vi "限幅器（Path）.vi"(3 "下限":path, 4 "X_in":path, 5 "上限":path) -> (1 "X_Out":path)   [LabVIEW 2012]
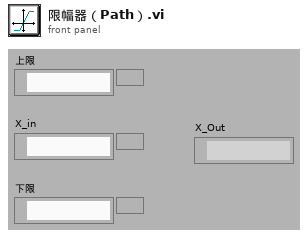
[diagram p1: front panel]
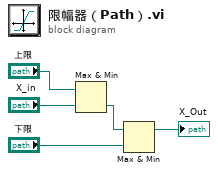
[diagram p0: block diagram]
diagram:
  n1 = Max & Min(x="上限", y="X_in") -> (min(x,y)=w3:path)  [unwired: 1 out]
  n2 = Max & Min(x=w3, y="下限") -> (max(x,y)=→"X_Out":path)  [unwired: 1 out]
